vi "GEA3 Set Mix Valve Position.vi"(6 "Disable Check":bool=TRUE, 8 "error in (no error)":errorcluster, 10 "MIX VALVE STEP OFFSET (0x400A)":i16, 11 ".NET Refnum in":refnum<k24>) -> (0 "error out":errorcluster, 1 "GEA Message":T1 {"Command" format="%02x"; "Destination" format="%02x"; "Source" format="%02x"}, 2 "Raw Data Out":string, 3 ".NET Refnum out":refnum<k24>, 5 "Initial Mix Valve Position":u16, 7 "Final Mix Valve Position":u16)   [LabVIEW 2019]
uses:
  type defs/Data In.ctl
  C:/TechnologyLab/NI-2010/Drivers/GEA3 Toolkit/GEA3 DLL Source/GeaCommunication.dll
  GEA3 DLL Source/GeaCommunication.dll
  type defs/ERD Write Data In.ctl
  type defs/Data Type.ctl
  library/GEA2_Toolkit.lvlib
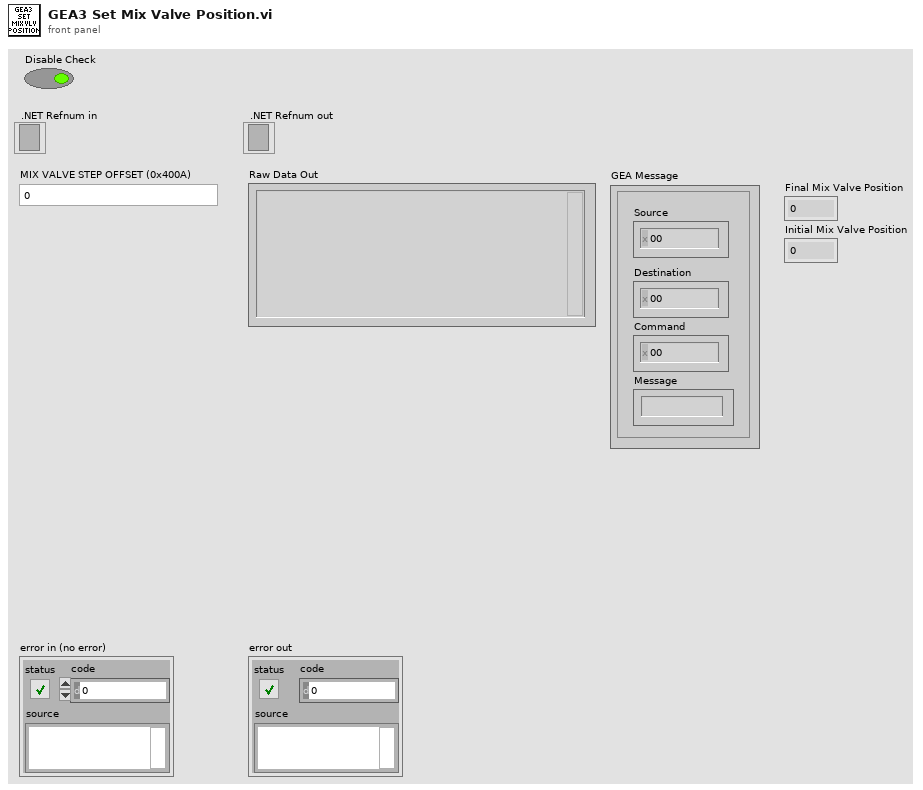
[diagram p1: front panel]
types:
  T1 = typedef "GEA2_Toolkit.lvlib/Data In.ctl" = cluster{"Source":u8, "Destination":u8, "Command":u8, "Message":string}
  T2 = typedef "GEA2_Toolkit.lvlib/ERD Write Data In.ctl" = cluster{"ERD Number":u16, "Data Type":T3, "Data":string}
  T3 = typedef "GEA2_Toolkit.lvlib/Data Type.ctl" = enum16{"string", "boolean", "uint8_t", "uint16_t", "uint32_t", "uint64_t", "int8_t", "int16_t", "int32_t", "int64_t"}
  T4 = typedef "GEA2_Toolkit.lvlib/Source_Destination.ctl" = cluster{"Source":u8, "Destination":u8}
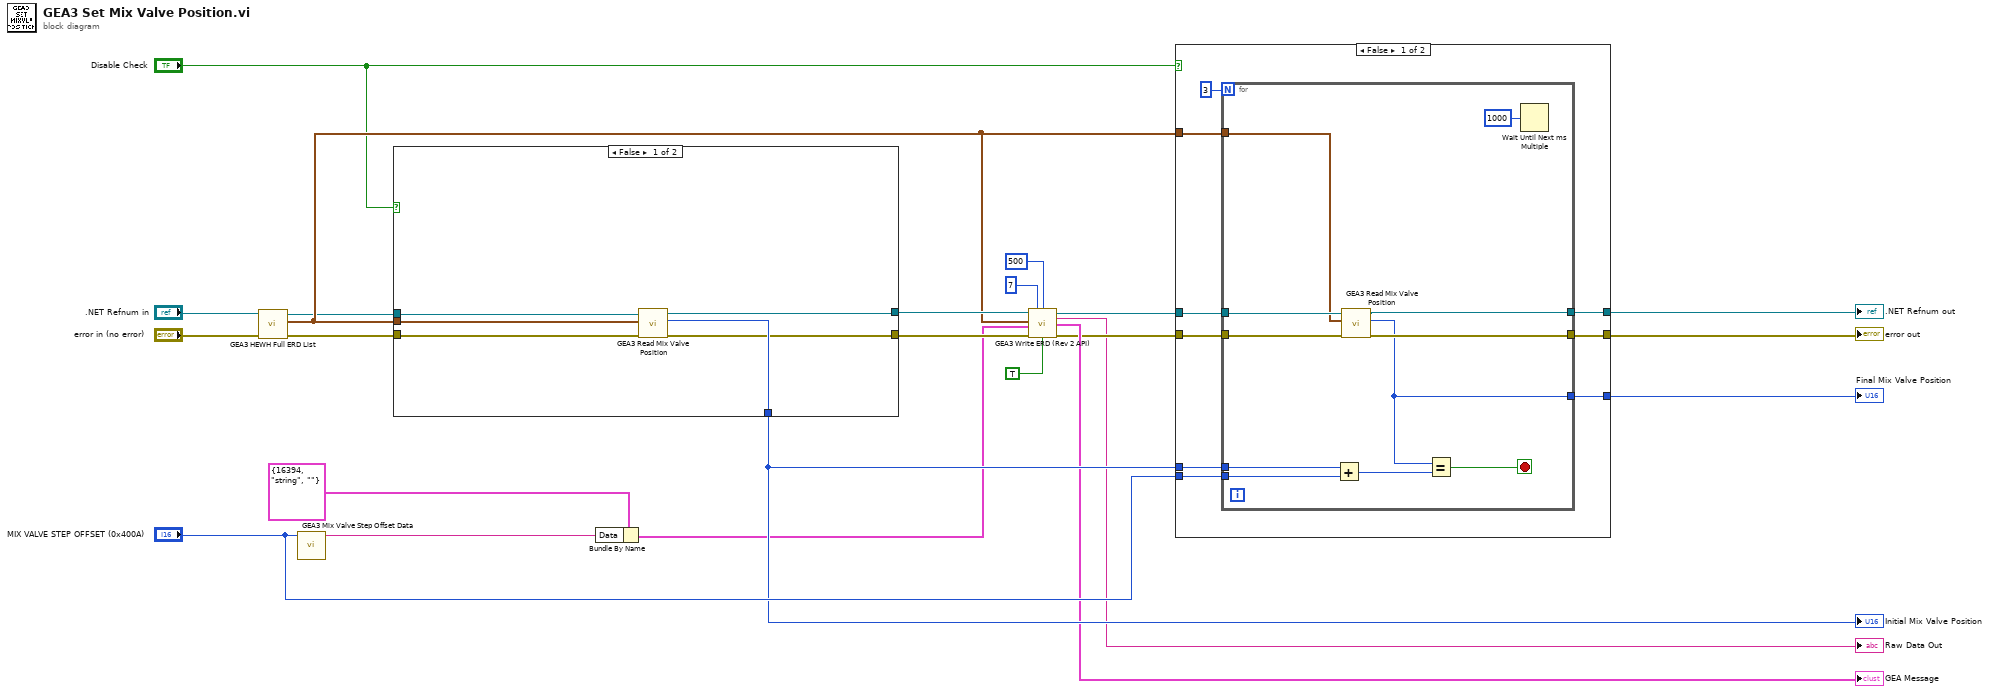
[diagram p0: block diagram]
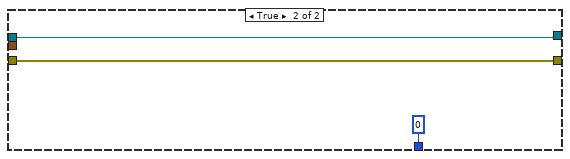
[diagram p2: hidden frame]
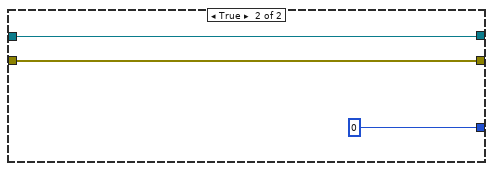
[diagram p3: hidden frame]
diagram:
  n1 = call "GEA3 HEWH Full ERD List.vi"("error in (no error)"="error in (no error)", "GEA2 Reference In"=".NET Refnum in") -> ("error out"=w15:errorcluster, "GEA Inputs"=w16:T4, "GEA2 Reference Out"=w14:refnum<k24>)  [unwired: 5 in, 2 out]
  n2 = call "GEA3 Mix Valve Step Offset Data.vi"("MIX VALVE STEP OFFSET (0x400A)"="MIX VALVE STEP OFFSET (0x400A)") -> ("Conv Message Out"=w10:string)  [unwired: 9 in, 1 out]
  n3 = case shown="False" "Disable Check" {
    tunnel: [w29 u16 0 ("Number Out")] -> w22
    tunnel: [w28 w31] -> w18
    tunnel: [w27 w32] -> w17
    tunnel: w16 -> [w26 _]
    tunnel: w15 -> [w25 w31]
    tunnel: w14 -> [w24 w32]
    frame False {
      n4 = call "GEA3 Read Mix Valve Position.vi"("error in (no error)"=w25, "GEA Inputs"=w26, ".NET Refnum in"=w24) -> ("error out"=w28:errorcluster, "Mix Valve Position"=w29:i16, ".NET Refnum out"=w27:refnum<k24>)  [unwired: 6 in]
    }
    frame True {
    }
  }
  "Initial Mix Valve Position" <- w22
  n5 = Bundle By Name(cluster=T2 {"ERD Number"=16394, "Data Type"=enum."string", "Data"=""} ("ERD Write Data In"), "Data"=w10) -> (w11:T2)
  n6 = call "GEA3 Write ERD (Rev 2 API).vi"("GEA2 Reference In"=w17, "# of Tries"=u8 7, "Read Timeout (ms)"=u32 500, "GEA Inputs"=w16, "ERD Write Data In"=w11, "Error In"=w18, "Verify ERD Response?"=TRUE) -> ("GEA2 Reference Out"=w7:refnum<k24>, "Raw Data Out"=→"Raw Data Out":string, "GEA Message"=→"GEA Message":T1, "Error Out"=w8:errorcluster)  [unwired: 5 in]
  n7 = case shown="False" "Disable Check" {
    tunnel: "MIX VALVE STEP OFFSET (0x400A)" -> [w41 _]
    tunnel: w22 -> [w40 _]
    tunnel: [w39 w54] -> w20
    tunnel: [w38 w55] -> w19
    tunnel: w16 -> [w36 _]
    tunnel: w8 -> [w35 w54]
    tunnel: w7 -> [w34 w55]
    tunnel: [w33 u16 0 ("Number Out")] -> w2
    frame False {
      n8 = for {
        N: 3 -> [_]
        tunnel: w34 -> [w47]
        tunnel: w35 -> [w48]
        tunnel: w36 -> [w43]
        tunnel: [w46] -> w38
        tunnel: [w45] -> w39
        tunnel: w40 -> [w52]
        tunnel: w41 -> [w51]
        tunnel: [w44] -> w33
        stop <- w49 stop-if-true
        n9 = Add(x=w52, y=w51) -> (x+y=w50:u16)
        n10 = call "GEA3 Read Mix Valve Position.vi"("error in (no error)"=w48, "GEA Inputs"=w43, ".NET Refnum in"=w47) -> ("error out"=w45:errorcluster, "Mix Valve Position"=w44:i16, ".NET Refnum out"=w46:refnum<k24>)  [unwired: 6 in]
        n11 = Equal?(x=w44, y=w50) -> (x = y?=w49:bool)
        n12 = Wait Until Next ms Multiple(millisecond multiple=u32 1000) -> ()  [unwired: 1 out]
      }
    }
    frame True {
    }
  }
  "error out" <- w20
  ".NET Refnum out" <- w19
  "Final Mix Valve Position" <- w2
